vi "Lift Zero Encoder.vi"   [LabVIEW 2014]
uses:
  Robot Global Data.vi
types:
  T1 = typedef "WPI_MotorControlDeviceRef.ctl" = cluster{"DeviceStatus":errorcluster, "Type":T2, "PWM":cluster{"Controller":T3, "PWM Channel":T4, "DeadBand":T5}, "CAN":cluster{"Device Number":u8, "Control Mode":T6, "Semaphore":T7, "Max Vout":dbl, "TalonSRX Control Mode":T8}, "Invert":bool, "TransformRef":T9, "InvTransformRef":T9}
  T2 = typedef "WPI_MotorControlType.ctl" = enum16{"PWM", "CAN", "CANTalonSRX"}
  T3 = typedef "FPGA_TypedefDigitalModule.ctl" = enum16{"Controller 1"}
  T4 = typedef "FPGA_DIOPWMChannel.ctl" = enum8{"PWM 0", "PWM 1", "PWM 2", "PWM 3", "PWM 4", "PWM 5", "PWM 6", "PWM 7", "PWM 8", "PWM 9", "PWM MXP 0", "PWM MXP 1", "PWM MXP 2", "PWM MXP 3", "PWM MXP 4", "PWM MXP 5", "PWM MXP 6", "PWM MXP 7", "PWM MXP 8", "PWM MXP 9", "Invalid"}
  T5 = typedef "WPI_PWMDeadband.ctl" = cluster{"Name":string, "maxPositivePwm":i32, "minPositivePwm":i32, "centerPwm":i32, "maxNegativePwm":i32, "minNegativePwm":i32, "angularRange":u16}
  T6 = typedef "WPI_CANJaguar_ControlMode.ctl" = enum8{"Percent VBus", "Current", "Speed", "Position", "Voltage"}
  T7 = typedef "Semaphore RefNum" = refnum<k1>
  T8 = typedef "WPI_CANTalonSRX_APIControlMode.ctl" = enum8{"Percent VBus", "Speed", "Position", "Slave", "Unchanged / Invalid"}
  T9 = typedef "WPI_PWMTransform_ConPane.ctl" = refnum<vi>
  T10 = typedef "WPI_EncoderDevRef.ctl" = cluster{"DevStatus":errorcluster, "EncoderIndex":T11, "CounterIndex":T12, "DistancePerCount":dbl, "Decoding Type":T13}
  T11 = typedef "FPGA_EncoderIdx.ctl" = enum8{"Enc 0", "Enc 1", "Enc 2", "Enc 3", "Enc 4", "Enc 5", "Enc 6", "Enc 7", "Invalid"}
  T12 = typedef "FPGA_CounterCtrSystemIndex.ctl" = enum8{"Ctr 0", "Ctr 1", "Ctr 2", "Ctr 3", "Ctr 4", "Ctr 5", "Ctr 6", "Ctr 7", "Invalid"}
  T13 = typedef "WPI_EncoderType.ctl" = enum16{"1x", "2x", "4x"}
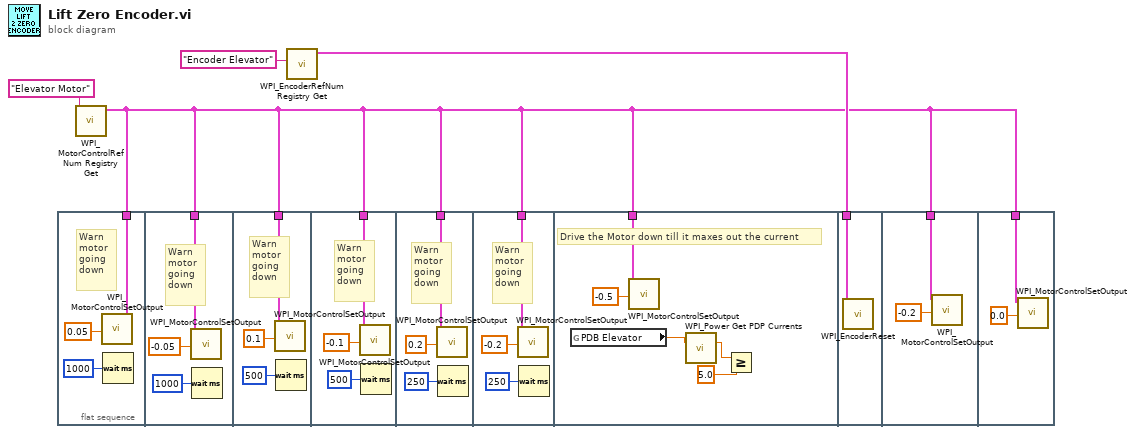
[diagram p0: block diagram]
diagram:
  n1 = flat-sequence {
    tunnel: w2 -> [w7]
    tunnel: w2 -> [w8]
    tunnel: w2 -> [w11]
    tunnel: w2 -> [w14]
    tunnel: w2 -> [w17]
    tunnel: w2 -> [w20]
    tunnel: w2 -> [w23]
    tunnel: w3 -> [w28]
    tunnel: w2 -> [w29]
    tunnel: w2 -> [w31]
    frame #0 {
      # "Warn \nmotor \ngoing \ndown"
      n2 = call <vilib>:"WPI_MotorControlSetOutput.vi"("Output"=0.05 ("y"), "MotorControlDevRef"=w7) -> ()  [unwired: 7 in, 3 out]
      n3 = Wait (ms)(milliseconds to wait=u32 1000) -> ()  [unwired: 1 out]
    }
    frame #1 {
      # "Warn \nmotor \ngoing \ndown"
      n4 = call <vilib>:"WPI_MotorControlSetOutput.vi"("Output"=-0.05 ("y"), "MotorControlDevRef"=w8) -> ()  [unwired: 7 in, 3 out]
      n5 = Wait (ms)(milliseconds to wait=u32 1000) -> ()  [unwired: 1 out]
    }
    frame #2 {
      # "Warn \nmotor \ngoing \ndown"
      n6 = call <vilib>:"WPI_MotorControlSetOutput.vi"("Output"=0.1 ("y"), "MotorControlDevRef"=w11) -> ()  [unwired: 7 in, 3 out]
      n7 = Wait (ms)(milliseconds to wait=u32 500) -> ()  [unwired: 1 out]
    }
    frame #3 {
      # "Warn \nmotor \ngoing \ndown"
      n8 = call <vilib>:"WPI_MotorControlSetOutput.vi"("Output"=-0.1 ("y"), "MotorControlDevRef"=w14) -> ()  [unwired: 7 in, 3 out]
      n9 = Wait (ms)(milliseconds to wait=u32 500) -> ()  [unwired: 1 out]
    }
    frame #4 {
      # "Warn \nmotor \ngoing \ndown"
      n10 = call <vilib>:"WPI_MotorControlSetOutput.vi"("Output"=0.2 ("y"), "MotorControlDevRef"=w17) -> ()  [unwired: 7 in, 3 out]
      n11 = Wait (ms)(milliseconds to wait=u32 250) -> ()  [unwired: 1 out]
    }
    frame #5 {
      # "Warn \nmotor \ngoing \ndown"
      n12 = call <vilib>:"WPI_MotorControlSetOutput.vi"("Output"=-0.2 ("y"), "MotorControlDevRef"=w20) -> ()  [unwired: 7 in, 3 out]
      n13 = Wait (ms)(milliseconds to wait=u32 250) -> ()  [unwired: 1 out]
    }
    frame #6 {
      # "Drive the Motor down till it maxes out the current"
      n14 = global read "Robot Global Data.vi" "PDB Elevator"() -> (w25:dbl)
      n15 = call <vilib>:"WPI_MotorControlSetOutput.vi"("Output"=-0.5 ("y"), "MotorControlDevRef"=w23) -> ()  [unwired: 7 in, 3 out]
      n16 = call <vilib>:"WPI_Power Get PDP Currents.vi"("PDP Channel"=w25) -> ("current (A)"=w26:dbl)  [unwired: 12 in, 2 out]
      n17 = Greater Or Equal?(x=w26, y=5.0) -> ()  [unwired: 1 out]
    }
    frame #7 {
      n18 = call <vilib>:"WPI_EncoderReset.vi"("EncoderDevRef"=w28) -> ()  [unwired: 9 in, 2 out]
    }
    frame #8 {
      n19 = call <vilib>:"WPI_MotorControlSetOutput.vi"("Output"=-0.2 ("y"), "MotorControlDevRef"=w29) -> ()  [unwired: 7 in, 3 out]
    }
    frame #9 {
      n20 = call <vilib>:"WPI_MotorControlSetOutput.vi"("Output"=0.0 ("y"), "MotorControlDevRef"=w31) -> ()  [unwired: 7 in, 3 out]
    }
  }
  n21 = call <vilib>:"WPI_MotorControlRefNum Registry Get.vi"("refnum name"="Elevator Motor") -> ("MotorControlDevRef"=w2:T1)  [unwired: 9 in, 1 out]
  n22 = call <vilib>:"WPI_EncoderRefNum Registry Get.vi"("refnum name"="Encoder Elevator") -> ("EncoderDevRef"=w3:T10)  [unwired: 9 in, 1 out]
